vi "ROI group-Get group setup by name.vi"(8 "error in":errorcluster, 11 "Name of ROI group to search for":string) -> (0 "error out (no error)":errorcluster, 1 "Found?":enum16{"Found", "Not found"}(ring), 3 "POI group info cluster":T1 {"Group region specifier cluster"."Contours"."Type" items=["No Selection", "Point", "Line", "Rectangle", "Oval", "Polygon", "Freehand Region", "Annulus", "Unused2", "Unused3", "Broken Line", "Freehand Line", "Rotated Rectangle"]})   [LabVIEW 2013]
uses:
  ROI Selection Interface/ROI group info cluster.ctl
  Typedefs/Get-Set-Clear Control.ctl
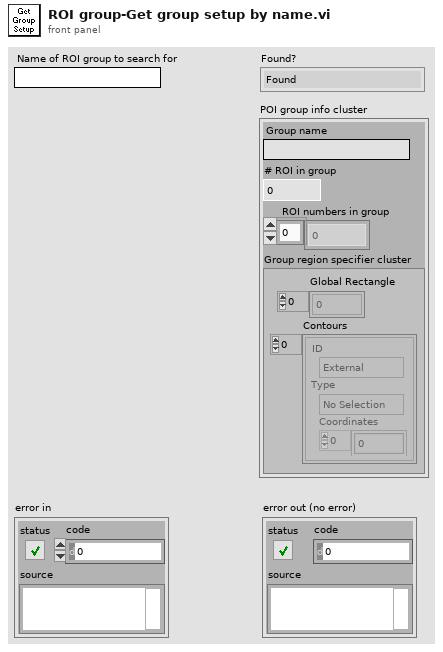
[diagram p1: front panel]
types:
  T1 = typedef "ROI group info cluster.ctl" = cluster{"Group name":string, "# ROI in group":i32, "ROI numbers in group":i32[], "Group region specifier cluster":T2}
  T2 = typedef "ROI Descriptor" = cluster{"Global Rectangle":i32[], "Contours":cluster{"ID":enum32{"External", "Internal"}, "Type":u32, "Coordinates":i32[]}[]}
  T3 = typedef "Get-Set-Clear Control.ctl" = enum16{"Get", "Set", "Clear"}
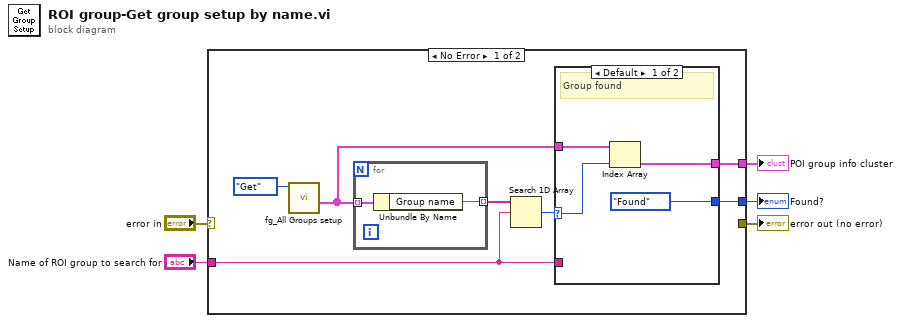
[diagram p0: block diagram]
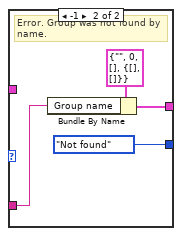
[diagram p2: hidden frame]
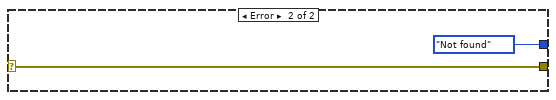
[diagram p3: hidden frame]
diagram:
  n1 = case shown="No Error" "error in" {
    selector: "error in" -> [_ w24]
    tunnel: [w12 enum16{"Found", "Not found"}."Not found" ("Found?")] -> w5
    tunnel: [w11 _] -> w4
    tunnel: "Name of ROI group to search for" -> [w8 _]
    tunnel: [_ w24] -> w1
    frame No Error {
      n2 = call "fg_All Groups setup.vi"("Function"=Get-Set-Clear_Control."Get") -> ("Groups setup out"=w6:T1[])  [unwired: 9 in, 1 out]
      n3 = for {
        tunnel: w6 -> [w22] mode=indexing
        tunnel: [w21] -> w9 mode=indexing
        n4 = Unbundle By Name(w22) -> ("Group name"=w21:string)
      }
      n5 = Search 1D Array(1D array=w9, element=w8) -> (index of element=w10:i32)  [unwired: 1 in]
      n6 = case shown="Default" w10 {
        selector: w10 -> [w15 _]
        tunnel: w6 -> [w16 _]
        tunnel: [w14 w18] -> w11
        tunnel: [enum16{"Found", "Not found"}."Found" ("Found?") enum16{"Found", "Not found"}."Not found" ("Found?")] -> w12
        tunnel: w8 -> [_ w17]
        frame Default {
          # "Group found"
          n7 = Index Array(array=w16, index=w15) -> (element=w14:T1)
        }
        frame -1 {
          # "Error. Group was not found by name."
          n8 = Bundle By Name(cluster=T1 {"Group name"="", "# ROI in group"=0, "ROI numbers in group"=[], "Group region specifier cluster"={"Global Rectangle"=[], "Contours"=[]}} ("POI group info cluster 2"), "Group name"=w17) -> (w18:T1)
        }
      }
    }
    frame Error {
    }
  }
  "Found?" <- w5
  "POI group info cluster" <- w4
  "error out (no error)" <- w1
